vi "Register Existing DBL Item.vi"(8 "error in (no error)":errorcluster, 9 "notifier in":refnum<notifier>, 10 "Tag Name":string, 11 "Current Value Table in":refnum<class "Current Value Table.lvclass">) -> (0 "error out":errorcluster, 3 "Current Value Table out":refnum<class "Current Value Table.lvclass">)   [LabVIEW 2024, in "Current Value Table.lvlib" / "Current Value Table.lvclass"]
uses:
  Current Value Table.lvclass
  CVT_DBL/CVT_DBL.lvclass
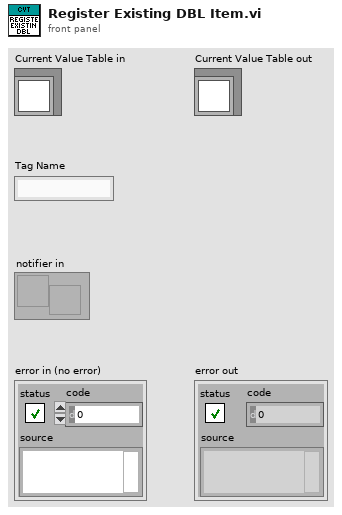
[diagram p1: front panel]
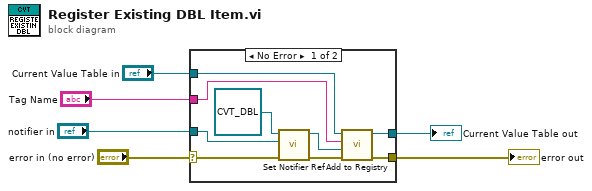
[diagram p0: block diagram]
diagram:
  n1 = case shown="No Error" "error in (no error)" {
    selector: "error in (no error)" -> [w14 w17]
    tunnel: [w9 w17] -> w5
    tunnel: [w11 w16] -> w3
    tunnel: "Current Value Table in" -> [w12 w16]
    tunnel: "notifier in" -> [w13 _]
    tunnel: "Tag Name" -> [w7 _]
    frame No Error {
      n2 = call-dynamic "Set Notifier Ref.vi"("error in (no error)"=w14, "notifier in"=w13, "CVT_DBL in"=refnum<class "CVT_DBL.lvclass"> refnum ("Current Value Table.lvlib:CVT_DBL.lvclass")) -> ("error out"=w10:errorcluster, "CVT_DBL out"=w8:refnum<class "CVT_DBL.lvclass">)  [unwired: 7 in]
      n3 = call-dynamic "Add to Registry.vi"("error in (no error)"=w10, "iCVT_Item in"=w8, "Tag Name"=w7, "Current Value Table in"=w12) -> ("error out"=w9:errorcluster, "Current Value Table out"=w11:refnum<class "Current Value Table.lvclass">)  [unwired: 5 in, 1 out]
    }
    frame Error {
    }
  }
  "error out" <- w5
  "Current Value Table out" <- w3
